vi "DeterminePropertyInterceptor.vi"(10 "Data name":string, 11 "Terminal in":refnum<vi>) -> (2 "interceptor":u32, 3 "arrayLevels":i32)   [LabVIEW 2013]
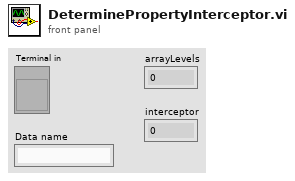
[diagram p1: front panel]
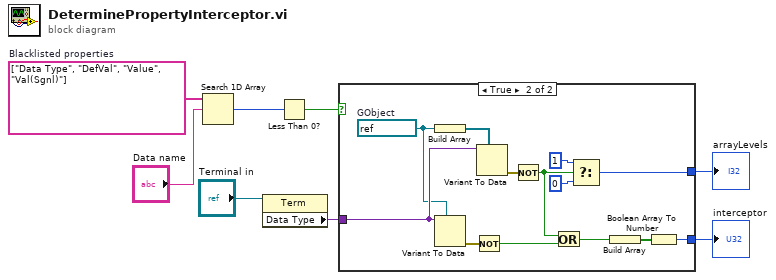
[diagram p0: block diagram]
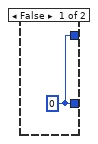
[diagram p2: hidden frame]
diagram:
  w3 = string[] ["Data Type", "DefVal", "Value", "Val(Sgnl)"]  # Blacklisted properties
  n1 = Search 1D Array(1D array=w3, element="Data name") -> (index of element=w2:i32)  [unwired: 1 in]
  n2 = property class="Term"(reference="Terminal in") -> ("Data Type"=w7:variant)  [unwired: 1 in, 2 out]
  n3 = Less Than 0?(x=w2) -> (x < 0?=w1:bool)
  n4 = case shown="True" w1 {
    tunnel: [w9 w15] -> w6
    tunnel: w7 -> [_ w14]
    tunnel: [w9 w11] -> w8
    frame False {
      w9 = 0 ("f")
    }
    frame True {
      w13 = refnum<vi> refnum  # GObject
      n5 = Build Array(w13) -> (w21:refnum<vi>[])
      n6 = Variant To Data(type=w13, Variant=w14) -> (error out=w22:errorcluster)  [unwired: 1 in, 1 out]
      n7 = Not(x=w22) -> (.not. x?=w19:bool)
      n8 = Variant To Data(type=w21, Variant=w14) -> (error out=w20:errorcluster)  [unwired: 1 in, 1 out]
      n9 = Not(x=w20) -> (.not. x?=w18:bool)
      n10 = Or(x=w18, y=w19) -> (x .or. y?=w12:bool)
      n11 = Select(t=1, s=w18, f=0) -> (s? t:f=w15:i32)
      n12 = Build Array(w12) -> (w10:bool[])
      n13 = Boolean Array To Number(Boolean array=w10) -> (number=w11:u32)
    }
  }
  "interceptor" <- w8
  "arrayLevels" <- w6
